vi "RANGE Create File Path.vi"(8 "Error In":errorcluster, 11 "File Path":string="C:\\Gas Flow Meter\\") -> (0 "Error Out":errorcluster, 3 "Path":path)   [LabVIEW 2019]
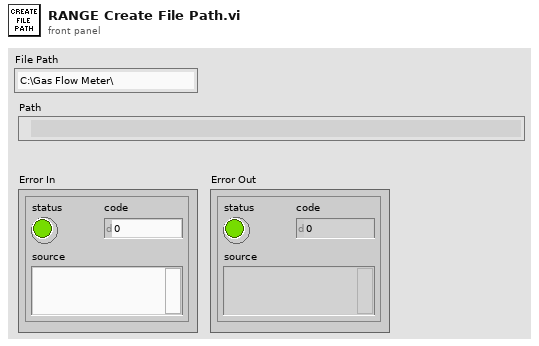
[diagram p1: front panel]
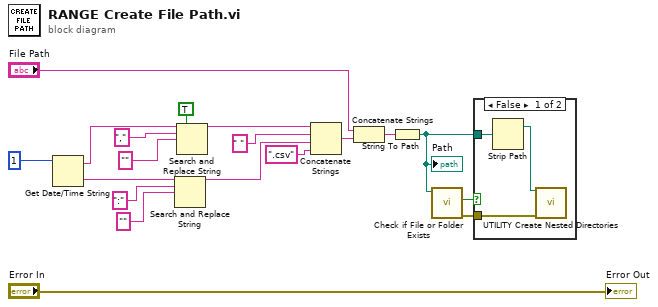
[diagram p0: block diagram]
diagram:
  n1 = Get Date/Time String(date format (0)=1) -> (date string=w12:string, time string=w9:string)  [unwired: 2 in]
  n2 = Search and Replace String(input string=w9, search string=":", replace string="") -> (result string=w17:string)  [unwired: 5 in, 3 out]
  n3 = Search and Replace String(replace all?=TRUE, input string=w12, search string=",", replace string="") -> (result string=w18:string)  [unwired: 4 in, 3 out]
  n4 = Concatenate Strings(w18, " ", w17, ".csv") -> (w4:string)
  n5 = Concatenate Strings("File Path", w4) -> (w5:string)
  n6 = String To Path(string=w5) -> (path=w2:path)
  "Path" <- w2
  n7 = call <vilib>:"Check if File or Folder Exists.vi"("path"=w2) -> ("error out"=w1:errorcluster, "file or folder exists?"=w3:bool)  [unwired: 8 in, 1 out]
  n8 = case shown="False" w3 {
    tunnel: w2 -> [w22 _]
    tunnel: w1 -> [w21 _]
    frame False {
      n9 = Strip Path(path=w22) -> (stripped path=w20:path)  [unwired: 1 out]
      n10 = call "UTILITY Create Nested Directories.vi"("path to create"=w20, "error in"=w21) -> ()  [unwired: 11 in, 3 out]
    }
    frame True {
    }
  }
  "Error Out" <- "Error In"
